vi "Get Transaction by Row.vi"(8 "error in (no error)":errorcluster, 10 "Row":u32, 11 "Credit Statement in":refnum<class "Credit Statement.lvclass">) -> (0 "error out":errorcluster, 2 "Transaction.lvclass":refnum<class "Transaction.lvclass">, 3 "Credit Statement out":refnum<class "Credit Statement.lvclass">)   [LabVIEW 2018]
uses:
  Statement/Statement.lvclass
  Transaction/Transaction.lvclass
  Credit Statement.lvclass
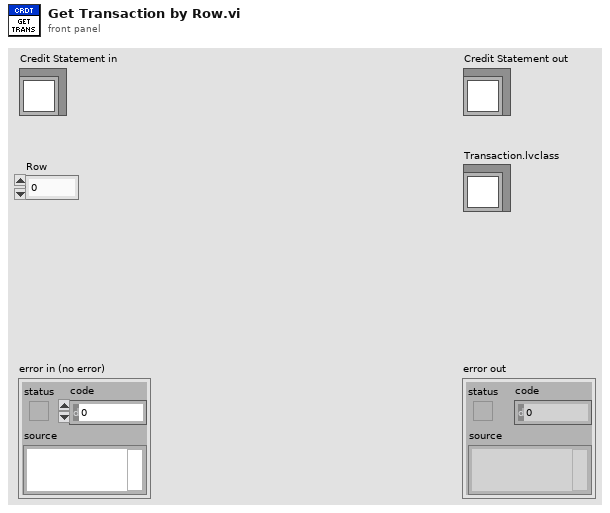
[diagram p1: front panel]
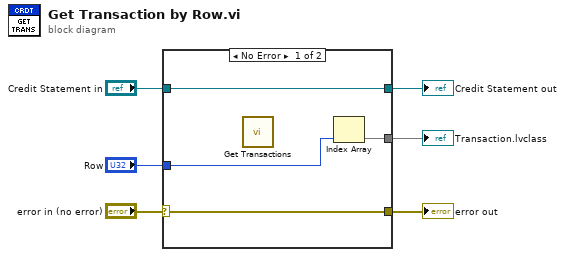
[diagram p0: block diagram]
diagram:
  n1 = case shown="No Error" "error in (no error)" {
    selector: "error in (no error)" -> [w8 w11]
    tunnel: "Credit Statement in" -> [w7 w12]
    tunnel: "Row" -> [w10 _]
    tunnel: [w9 _] -> w4
    tunnel: [w7 w12] -> w3
    tunnel: [w8 w11] -> w2
    frame No Error {
      n2 = call "Get Transactions.vi"() -> ()  [unwired: 9 in, 3 out]
      n3 = Index Array(index=w10) -> (element=w9)  [unwired: 1 in]
    }
    frame Error {
    }
  }
  "error out" <- w2
  "Credit Statement out" <- w3
  "Transaction.lvclass" <- w4
